vi "Unistat Generate Single Command Standalone.vi"(7 "Commands":string(combo)="Setup", 8 "error in (no error)":errorcluster, 9 "VISA resource":refnum<visa-resource-name>="COM1", 10 "Temperature":i32, 11 "Data Cluster":T1={"Current DoE"=[], "SSI 1 Flow Rate"=0.0, "SSI 2 Flow Rate"=0.0, "FLOM 1 Flow Rate"=0.0, "FLOM 2 Flow Rate"=0.0, "Pumps Running?"=FALSE, "Boolean 2"=FALSE, "Boolean 3"=FALSE, "Boolean 4"=FALSE, "At Equilibrium?"=FALSE, "Script Running?"=FALSE, "Current Script Iteration"=0.0, "Total Script Iterations"=0.0, "FLOM Pumps VISA"="COM2", "SSI 1 Pump VISA"="COM76", "SSI 2 Pump VISA"="COM74", "Huber Unistat VISA"="COM1", "SSI 3 Pump VISA"="COM76", "SSI 4 Pump VISA"="COM76", "SSI 4 Flow Rate"=0.0, "SSI 3 Flow Rate"=0.0, "Flow Meter 1"="COM76", "Flow Meter 2"="COM76", "Flow Meter 3"="COM76", "Flow Meter 4"="COM76", "Flow Meter 1 Rate "=0.0, "Flow Meter 2 Rate"=0.0, "Flow Meter 3 Rate"=0.0, "Flow Meter 4 Rate"=0.0, "SSI 1 Flow Setpoint"=0.0, "SSI 2 Flow Setpoint"=0.0, "SSI 3 Flow Setpoint"=0.0, "SSI 4 Flow Setpoint"=0.0, "Temperature Setpoint"=0.0} {"Current DoE" format="%0.3f"}) -> (0 "Error Out":T2, 1 "Temperature Output":string="Upper limit is", 2 "Last Message from Pump":string="Heating pump message, 2:38:53 PM:\nTemperature is set to 0.000000K", 3 "Data Cluster 2":T1={"Current DoE"=[], "SSI 1 Flow Rate"=0.0, "SSI 2 Flow Rate"=0.0, "FLOM 1 Flow Rate"=0.0, "FLOM 2 Flow Rate"=0.0, "Pumps Running?"=FALSE, "Boolean 2"=FALSE, "Boolean 3"=FALSE, "Boolean 4"=FALSE, "At Equilibrium?"=FALSE, "Script Running?"=FALSE, "Current Script Iteration"=0.0, "Total Script Iterations"=0.0, "FLOM Pumps VISA"="COM2", "SSI 1 Pump VISA"="COM76", "SSI 2 Pump VISA"="COM74", "Huber Unistat VISA"="COM1", "SSI 3 Pump VISA"="COM76", "SSI 4 Pump VISA"="COM76", "SSI 4 Flow Rate"=0.0, "SSI 3 Flow Rate"=0.0, "Flow Meter 1"="COM76", "Flow Meter 2"="COM76", "Flow Meter 3"="COM76", "Flow Meter 4"="COM76", "Flow Meter 1 Rate "=0.0, "Flow Meter 2 Rate"=0.0, "Flow Meter 3 Rate"=0.0, "Flow Meter 4 Rate"=0.0, "SSI 1 Flow Setpoint"=0.0, "SSI 2 Flow Setpoint"=0.0, "SSI 3 Flow Setpoint"=0.0, "SSI 4 Flow Setpoint"=0.0, "Temperature Setpoint"=0.0} {"Current DoE" format="%0.3f"}, 5 "Last Command Written":string="Upper limit is")   [LabVIEW 2015]
uses:
  --Controls and TypeDefs--/DoE_Control_Cluster.ctl
  <vilib>/Instr/_visa.llb/VISA Configure Serial Port (Instr).vi
panel:
  in  "bytes to read 2":u32=40
  # "Tested and Works as of 7/15/2014!"
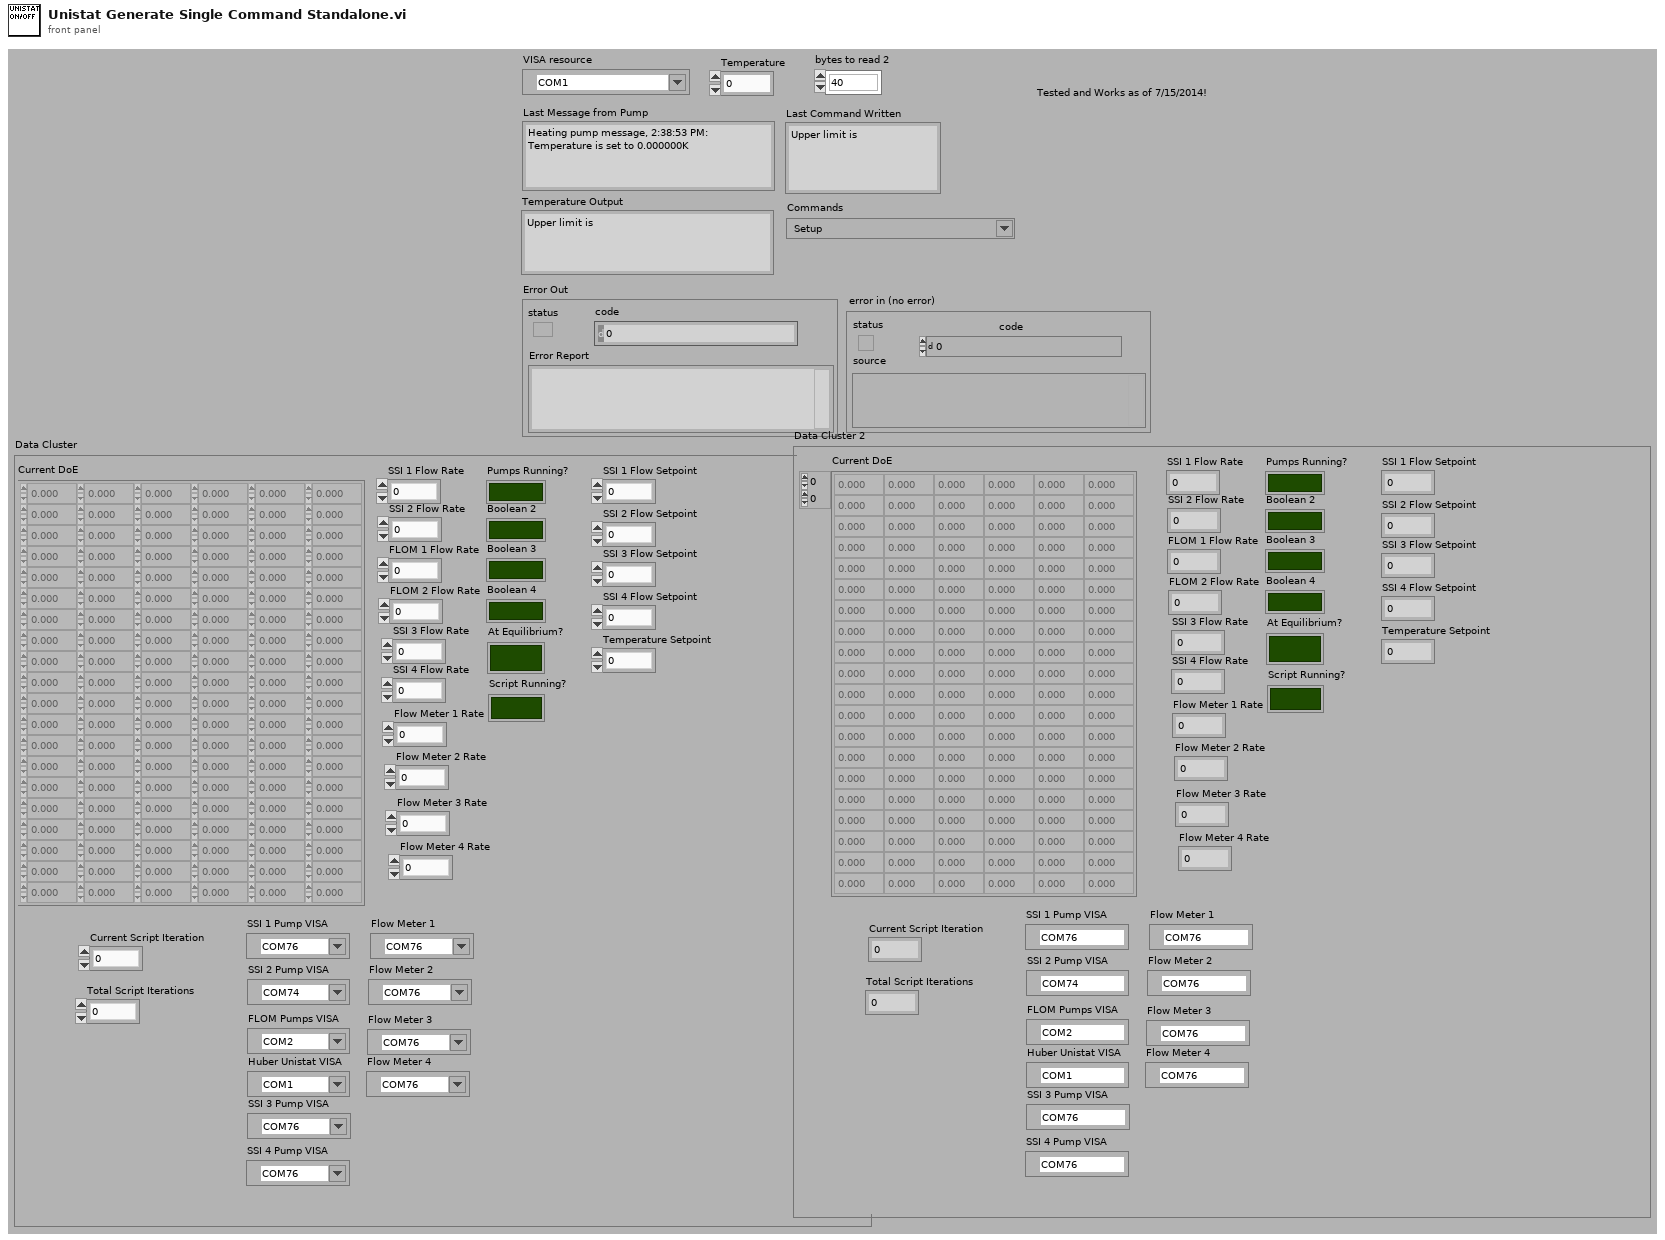
[diagram p1: front panel]
types:
  T1 = typedef "DoE_Control_Cluster.ctl" = cluster{"Current DoE":dbl[][], "SSI 1 Flow Rate":dbl, "SSI 2 Flow Rate":dbl, "FLOM 1 Flow Rate":dbl, "FLOM 2 Flow Rate":dbl, "Pumps Running?":bool, "Boolean 2":bool, "Boolean 3":bool, "Boolean 4":bool, "At Equilibrium?":bool, "Script Running?":bool, "Current Script Iteration":dbl, "Total Script Iterations":dbl, "FLOM Pumps VISA":refnum<visa-resource-name>, "SSI 1 Pump VISA":refnum<visa-resource-name>, "SSI 2 Pump VISA":refnum<visa-resource-name>, "Huber Unistat VISA":refnum<visa-resource-name>, "SSI 3 Pump VISA":refnum<visa-resource-name>, "SSI 4 Pump VISA":refnum<visa-resource-name>, "SSI 4 Flow Rate":dbl, "SSI 3 Flow Rate":dbl, "Flow Meter 1":refnum<visa-resource-name>, "Flow Meter 2":refnum<visa-resource-name>, "Flow Meter 3":refnum<visa-resource-name>, "Flow Meter 4":refnum<visa-resource-name>, "Flow Meter 1 Rate ":dbl, "Flow Meter 2 Rate":dbl, "Flow Meter 3 Rate":dbl, "Flow Meter 4 Rate":dbl, "SSI 1 Flow Setpoint":dbl, "SSI 2 Flow Setpoint":dbl, "SSI 3 Flow Setpoint":dbl, "SSI 4 Flow Setpoint":dbl, "Temperature Setpoint":dbl}
  T2 = cluster{"status":bool, "code":i32, "Error Report":string}
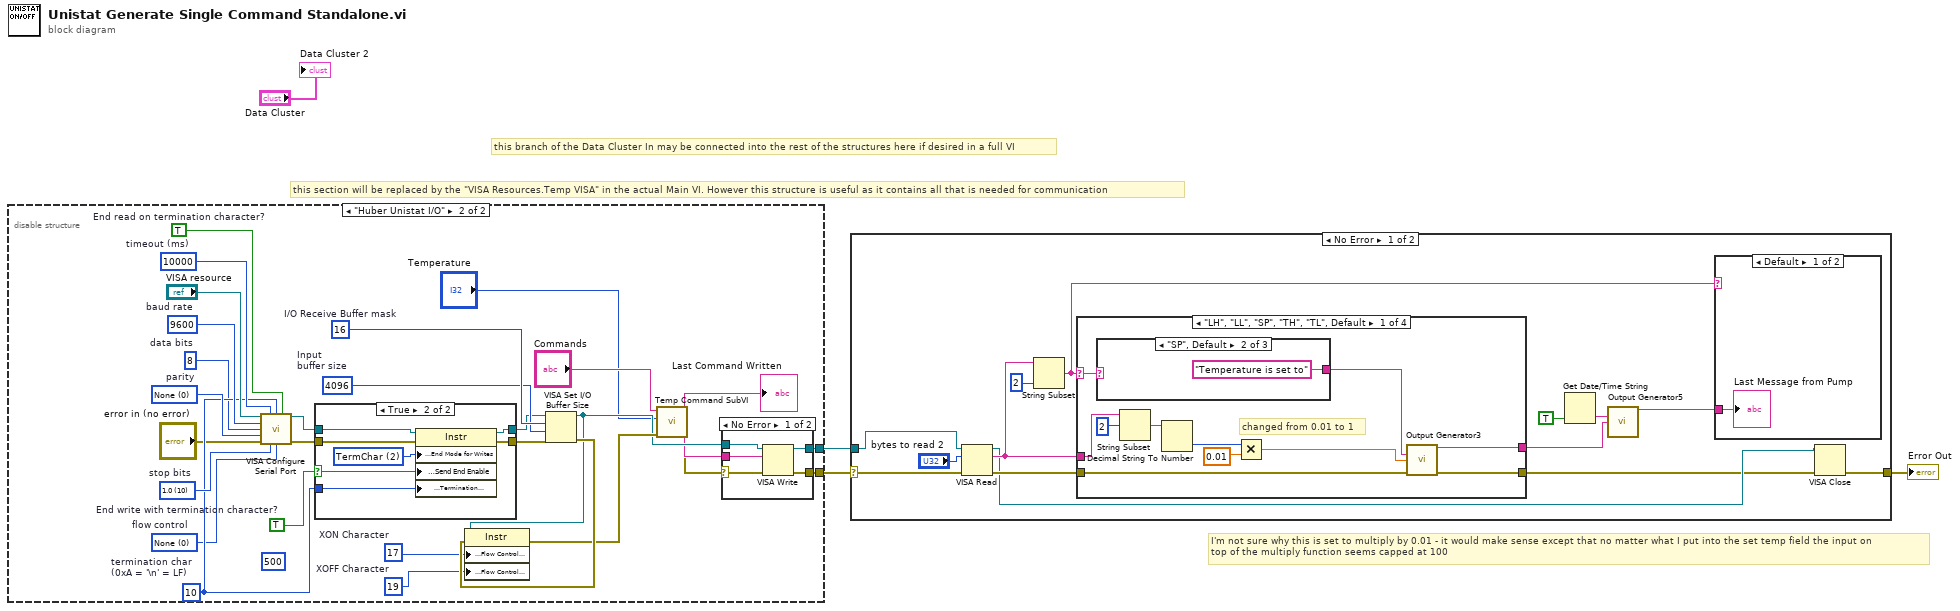
[diagram p0: block diagram]
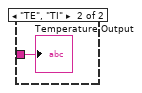
[diagram p5: hidden frame]
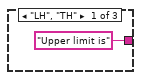
[diagram p6: hidden frame]
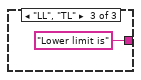
[diagram p7: hidden frame]
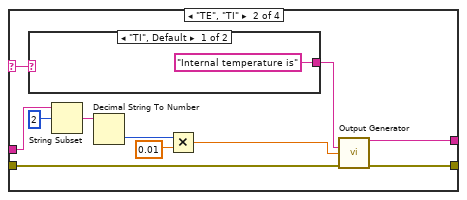
[diagram p8: hidden frame]
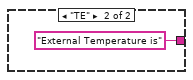
[diagram p9: hidden frame]
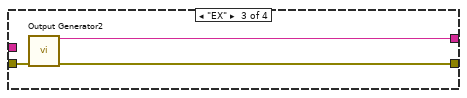
[diagram p10: hidden frame]
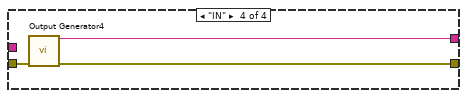
[diagram p11: hidden frame]
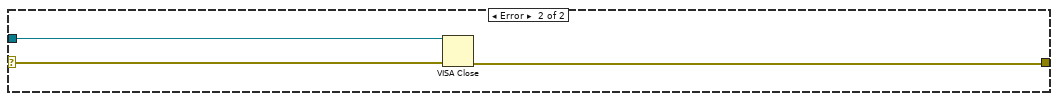
[diagram p12: hidden frame]
diagram:
  # "I'm not sure why this is set to multiply by 0.01 - it would make sense except that no matter what I put into the set temp field the input on\ntop of the multiply function seems capped at 100"
  # "this branch of the Data Cluster In may be connected into the rest of the structures here if desired in a full VI"
  # "this section will be replaced by the \"VISA Resources.Temp VISA\" in the actual Main VI. However this structure is useful as it contains all that is needed for communication"
  n1 = disable-structure shown="\"Huber Unistat I/O\"" {
    disable-tunnel: [_ w7] -> w3
    disable-tunnel: [_ w6] -> w2
    frame condition #0 {
    }
    frame condition #1 (active) {
      (unwired) 500
      w25 = u32 4096  # Input buffer size
      w19 = u8 19  # XOFF Character
      w20 = u8 17  # XON Character
      w28 = u32 10000  # timeout (ms)
      w27 = TRUE  # End read on termination character?
      w24 = TRUE  # End write with termination character?
      w23 = u8 10  # termination char (0xA = '\n' = LF)
      w22 = u16 0 items=["None"=0, "XON/XOFF"=1, "RTS/CTS"=2, "DTR/DSR"=4]  # flow control
      w29 = u16 10 items=["1.0"=10, "1.5"=15, "2.0"=20]  # stop bits
      w30 = u16 0 items=["None", "Odd", "Even", "Mark", "Space"]  # parity
      w18 = u16 8  # data bits
      w32 = u32 9600  # baud rate
      w26 = u16 16  # I/O Receive Buffer mask
      n2 = call-poly "VISA Configure Serial Port"("VISA resource name"="VISA resource", "timeout (10sec)"=w28, "termination char\n(0xA = '\\n' = LF)"=w23, "Enable Termination\nChar (T)"=w27, "baud rate (9600)"=w32, "data bits (8)"=w18, "parity (0:none)"=w30, "error in (no error)"="error in (no error)", "stop bits (10: 1 bit)"=w29, "flow control (0:none)"=w22) -> ("VISA resource name out"=w15:refnum<visa-resource-name>, "error out"=w17:errorcluster)  [unwired: 4 out]
      n3 = case shown="True" w24 {
        selector: w24 -> [_ w42]
        tunnel: w15 -> [w40 w48]
        tunnel: w17 -> [w41 w47]
        tunnel: [w40 w46] -> w13
        tunnel: [w41 w45] -> w16
        tunnel: w23 -> [_ w43]
        frame False {
        }
        frame True {
          w44 = u16 2 items=["None", "LastBit", "TermChar", "Break"] ("Serial Settings:Serial End Mode for Writes")
          n4 = property class="Instr"(reference=w48, error in=w47, "Serial Settings:End Mode for Writes"=w44, "Message Based Settings:Send End Enable"=w42, "Message Based Settings:Termination Character"=w43) -> (reference out=w46:refnum<visa-resource-name>, error out=w45:errorcluster)
        }
      }
      n5 = VISA Set I/O Buffer Size(VISA resource name=w13, mask (16)=w26, size (4096)=w25, error in (no error)=w16) -> (VISA resource name out=w11:refnum<visa-resource-name>, error out=w21:errorcluster)
      n6 = property class="Instr"(reference=w11, error in=w21, "Serial Settings:Flow Control XON Character"=w20, "Serial Settings:Flow Control XOFF Character"=w19) -> (error out=w12:errorcluster)  [unwired: 1 out]
      n7 = call "Temp Command SubVI.vi"("error in (no error)"=w12, "Numeric"="Temperature", "Commands"="Commands") -> ("error out"=w9:errorcluster, "Command String"=w10:string)  [unwired: 6 in]
      "Last Command Written" <- w10
      n8 = case shown="No Error" w9 {
        selector: w9 -> [w34 w38]
        tunnel: w11 -> [w36 w39]
        tunnel: w10 -> [w37 _]
        tunnel: [w33 w38] -> w6
        tunnel: [w35 w39] -> w7
        frame No Error {
          n9 = VISA Write(VISA resource name=w36, write buffer=w37, error in (no error)=w34) -> (VISA resource name out=w35:refnum<visa-resource-name>, error out=w33:errorcluster)  [unwired: 1 out]
        }
        frame Error {
        }
      }
    }
  }
  n10 = case "Read bytes from port." shown="No Error" w2 {
    selector: w2 -> [w60 w99]
    tunnel: [w49 w98] -> w4
    tunnel: w3 -> [w61 w100]
    frame No Error {
      n11 = VISA Read(VISA resource name=w61, byte count="bytes to read 2", error in (no error)=w60) -> (VISA resource name out=w51:refnum<visa-resource-name>, read buffer=w58:string, error out=w57:errorcluster)  [unwired: 1 out]
      n12 = String Subset(string=w58, length (rest)=2) -> (substring=w52:string)  [unwired: 1 out]
      n13 = case shown="\"LH\", \"LL\", \"SP\", \"TH\", \"TL\", Default" w52 {
        selector: w52 -> [w71 w86 _ _]
        tunnel: [w65 w87 w94 w95] -> w54
        tunnel: w58 -> [w73 w81 _ _]
        tunnel: [w74 w89 w92 w96] -> w50
        tunnel: w57 -> [w75 w88 w93 w97]
        frame "LH", "LL", "SP", "TH", "TL", Default {
          # "changed from 0.01 to 1"
          n14 = case shown="\"SP\", Default" w71 {
            tunnel: ["Upper limit is" "Temperature is set to" "Lower limit is"] -> w70
            frame "LH", "TH" {
            }
            frame "SP", Default {
            }
            frame "LL", "TL" {
            }
          }
          n15 = String Subset(string=w73, offset (0)=2) -> (substring=w69:string)  [unwired: 1 out]
          n16 = Decimal String To Number(string=w69) -> (number=w68:i32)  [unwired: 3 out]
          n17 = Multiply(x=w68, y=0.01) -> (x*y=w66:dbl)
          n18 = call "Output Generator3"("Query"=w70, "number"=w66, "error in (no error)"=w75) -> ("Result"=w65:string, "error out"=w74:errorcluster)  [unwired: 2 in, 9 out]
        }
        frame "TE", "TI" {
          n19 = case shown="\"TI\", Default" w86 {
            tunnel: ["Internal temperature is" "External Temperature is"] -> w79
            frame "TI", Default {
            }
            frame "TE" {
            }
          }
          n20 = String Subset(string=w81, offset (0)=2) -> (substring=w84:string)  [unwired: 1 out]
          n21 = Decimal String To Number(string=w84) -> (number=w83:i32)  [unwired: 3 out]
          n22 = Multiply(x=w83, y=0.01) -> (x*y=w80:dbl)
          n23 = call "Output Generator"("Query"=w79, "temp"=w80, "error in (no error)"=w88) -> ("Result"=w87:string, "error out"=w89:errorcluster)  [unwired: 2 in, 9 out]
        }
        frame "EX" {
          n24 = call "Output Generator2"("error in (no error)"=w93) -> ("Result"=w94:string, "error out"=w92:errorcluster)  [unwired: 2 in, 11 out]
        }
        frame "IN" {
          n25 = call "Output Generator4"("error in (no error)"=w97) -> ("Result"=w95:string, "error out"=w96:errorcluster)  [unwired: 2 in, 11 out]
        }
      }
      n26 = Get Date/Time String(want seconds? (F)=TRUE) -> (time string=w55:string)  [unwired: 3 out]
      n27 = call "Output Generator5"("Time"=w55, "Error Output"=w54) -> ("Result"=w53:string)  [unwired: 3 in, 10 out]
      n28 = case shown="Default" w52 {
        tunnel: w53 -> [w63 w64]
        frame Default {
          "Last Message from Pump" <- w63
        }
        frame "TE", "TI" {
          "Temperature Output" <- w64
        }
      }
      n29 = VISA Close(VISA resource name=w51, error in (no error)=w50) -> (error out=w49:errorcluster)
    }
    frame Error {
      n30 = VISA Close(VISA resource name=w100, error in (no error)=w99) -> (error out=w98:errorcluster)
    }
  }
  "Error Out" <- w4
  "Data Cluster 2" <- "Data Cluster"
